vi "Configure List Sweep.vi"(5 "Sweep Function A (0: Frequency)":u16(ring) items=["Frequency", "Voltage", "Current", "Bias Voltage", "Bias Current", "DC Source Voltage"], 7 "Sweep Function B (0: None)":u16(ring) items=["None", "Impedance Range", "Frequency", "Voltage", "Current", "Bias Voltage", "Bias Current", "DC Source Voltage"], 8 "error in (no error)":errorcluster, 9 "Sweep Mode (0: Sequence)":u16(ring) items=["Sequence", "Stepped"], 10 "Sweep Point Array":dbl[](array[numeric])=[0.0, 0.0, 0.0, 0.0, 0.0], 11 "Agilent 428x in":refnum<class "Agilent 428x.lvclass">) -> (0 "error out":errorcluster, 3 "Agilent 428x out":refnum<class "Agilent 428x.lvclass">)   [LabVIEW 2020, in "Agilent 428x.lvclass"]
uses:
  Agilent 428x.lvclass
  C:/Sandbox/Git_Sandbox/WiSpry Test Framework source code (LV20)/WiSpry Test Framework/Instruments/Instrument.lvclass
  Instrument.lvclass/Instrument.ctl
  Instrument.lvclass
  <instrlib>/Agilent 428X Series/Agilent 428X Series.lvlib
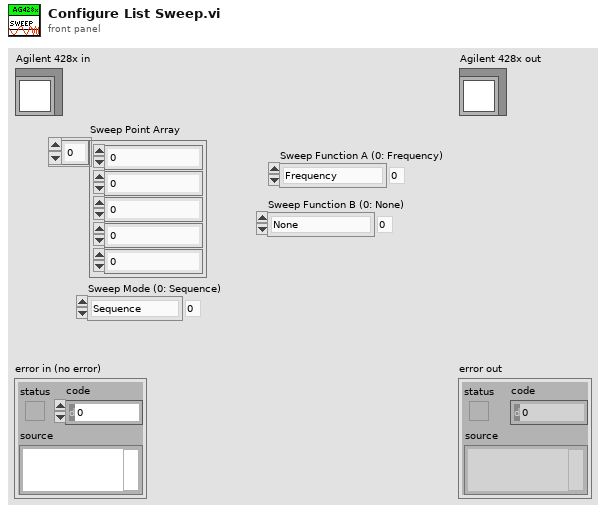
[diagram p1: front panel]
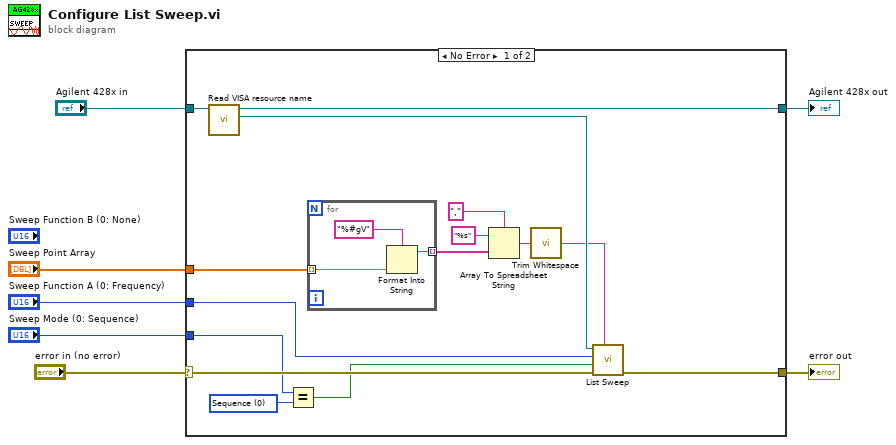
[diagram p0: block diagram]
diagram:
  n1 = case shown="No Error" "error in (no error)" {
    selector: "error in (no error)" -> [w19 w27]
    tunnel: [w18 w27] -> w6
    tunnel: [w21 w26] -> w5
    tunnel: "Agilent 428x in" -> [w22 w26]
    tunnel: "Sweep Function A (0: Frequency)" -> [w17 _]
    tunnel: "Sweep Mode (0: Sequence)" -> [w15 _]
    tunnel: "Sweep Point Array" -> [w9 _]
    frame No Error {
      w16 = u16 0 items=["Sequence", "Stepped"] ("Sweep Mode (0: Sequence)")
      n2 = call "Read VISA resource name.vi"("Instrument in"=w22) -> ("VISA resource name"=w20:refnum<visa-resource-name>, "Instrument out"=w21:refnum<class "Agilent 428x.lvclass">)  [unwired: 9 in]
      n3 = Equal?(x=w15, y=w16) -> (x = y?=w14:bool)
      n4 = for {
        tunnel: w9 -> [w24] mode=indexing
        tunnel: [w23] -> w13 mode=indexing
        n5 = Format Into String(format string="%#gV", w24) -> (resulting string=w23:string)  [unwired: 2 in, 1 out]
      }
      n6 = Array To Spreadsheet String(delimiter (Tab)=",", array=w13, 3:"%s" ("format string")) -> (spreadsheet string=w10:string)
      n7 = call <vilib>:"Trim Whitespace.vi"("string"=w10) -> ("trimmed string"=w8:string)  [unwired: 1 in]
      n8 = call <instrlib>:"List Sweep.vi"("Sweep Points Value"=w8, "error in (no error)"=w19, "Sweep Mode (T: Sequence)"=w14, "List Function (0: Frequency)"=w17, "VISA resource name"=w20) -> ("error out"=w18:errorcluster)  [unwired: 5 in, 1 out]
    }
    frame Error {
    }
  }
  "error out" <- w6
  "Agilent 428x out" <- w5
